vi "reg_check.vi"() -> ()   [LabVIEW 2019]
uses:
  Heating/ctl/ZY_control.ctl
  ctl/Z_State.ctl
  ctl/Y_state.ctl
  Heating/ctl/Z_State.ctl
  Heating/ctl/TMP_val.ctl
  Inputs/Ctl/Parameter State.ctl
  Alarms/Ctl/ALRs_State.ctl
  Alarms/Ctl/ALR_ON_OFF.ctl
  Alarms/Ctl/ALR_Parameters.ctl
  Alarms/Ctl/ALR code.ctl
  Alarms/Ctl/ALR type.ctl
  ctl/ZY_state_short.ctl
  ctl/Z.ctl
  Heating/ctl/Y_source.ctl
  ctl/Y_short.ctl
  ctl/Y_source.ctl
  Inputs/Ctl/Parameter State short.ctl
  Alarms/Ctl/ALR_Status_short.ctl
  ctl/control param.ctl
  projects/Additivs/Regulators/PROG/GM1_201007/HT1/HT1_ALR_on.vi
  Alarms/ALR select.vi
  Alarms/ALR RESETs.vi
  Alarms/ALR ON_OFFs.vi
  bronkhorst_Z.vi
  Heating/Z_switch_heating.vi
  Z_State_reg.vi
  Sequence/State1.vi
  Trigers/RS.vi
  Timer Delay/Timer.vi
  bronkhorst_reg.vi
  Heating/Heating.lvlib
  Alarms/Alarms.lvlib
  Inputs/Inputs.lvlib
  control.lvlib
panel:
  in  "Z_HSw":u32=2
  in  "Y_ASetState":T1=enum."auto"
  out "YB":bool
  out "ALR_L1":bool
  out "Y":dbl format="%.2f"
  out "ZY_State":T2={"Z"={"Z_Source"=enum."initialize", "Z_SetState"=enum."initialization", "Z_State"=enum."initialization", "Z_State_T"=0, "ALR  L1"=FALSE, "ALR  L2"=FALSE, "HH_run"=0}, "Y"={"Y_Source"=enum."initialize", "Y_SetState"=enum."initialize", "SP_Set"=0.0, "SP"=0.0, "PV"=0.0, "PV_State"={"code"=0, "visible"=FALSE, "color"=0}, "Y_preSet"=0.0, "Y_Set"=0.0, "Y"=0.0, "Y_State"={"code"=0, "visible"=FALSE, "color"=0}, "YB"=FALSE}, "ALR_Status"=[], "control param"={"proportional gain (Kc)"=1.0, "integral time (Ti, s)"=10.0, "derivative time (Td, s)"=1.0, "output high"=100.0, "output high start"=40.0, "output high stop"=40.0, "alr value"=0.0, "output low"=0.0, "output rate (EGU/s)"=5.0, "setpoint max"=100.0, "setpoint rate (EGU/min)"=10.0, "stop rate (EGU/min)"=5.0}} {"control param"."setpoint max" format="%.2f"; "control param"."stop rate (EGU/min)" min=0.001 format="%.2f"; "control param"."setpoint rate (EGU/min)" min=0.001 format="%.2f"; "control param"."output high stop" format="%.2f"; "control param"."output high start" format="%.2f"; "control param"."output rate (EGU/s)" min=0.001 format="%.2f"; "control param"."output low" format="%.2f"; "control param"."alr value" format="%.2f"; "control param"."output high" format="%.2f"; "control param"."derivative time (Td, s)" format="%.3f"; "control param"."integral time (Ti, s)" format="%.3f"; "control param"."proportional gain (Kc)" format="%.3f"; "Y"."Y" format="%.2f"; "Y"."Y_preSet" format="%.2f"; "Y"."SP" step=0.01 format="%.2f"; "Y"."Y_Set" format="%.2f"; "Y"."PV" step=0.01 format="%.2f"; "Y"."SP_Set" step=0.01 format="%.2f"}
  in  "TMP_val":T11
  in  "Z_ASetState":T5
  in  "ALR_ON_OFF 2":T18
  in  "ZY_control":T19={"Z_HSw"=2, "Z_HSetState"=enum."initialization", "Y_HSw"=2, "Y_HSetState"=enum."initialize", "SP"=0.0, "Y_H"=0.0, "Reset_ALR"=FALSE} {"Y_H" step=1.0; "SP" step=0.01 format="%.2f"}
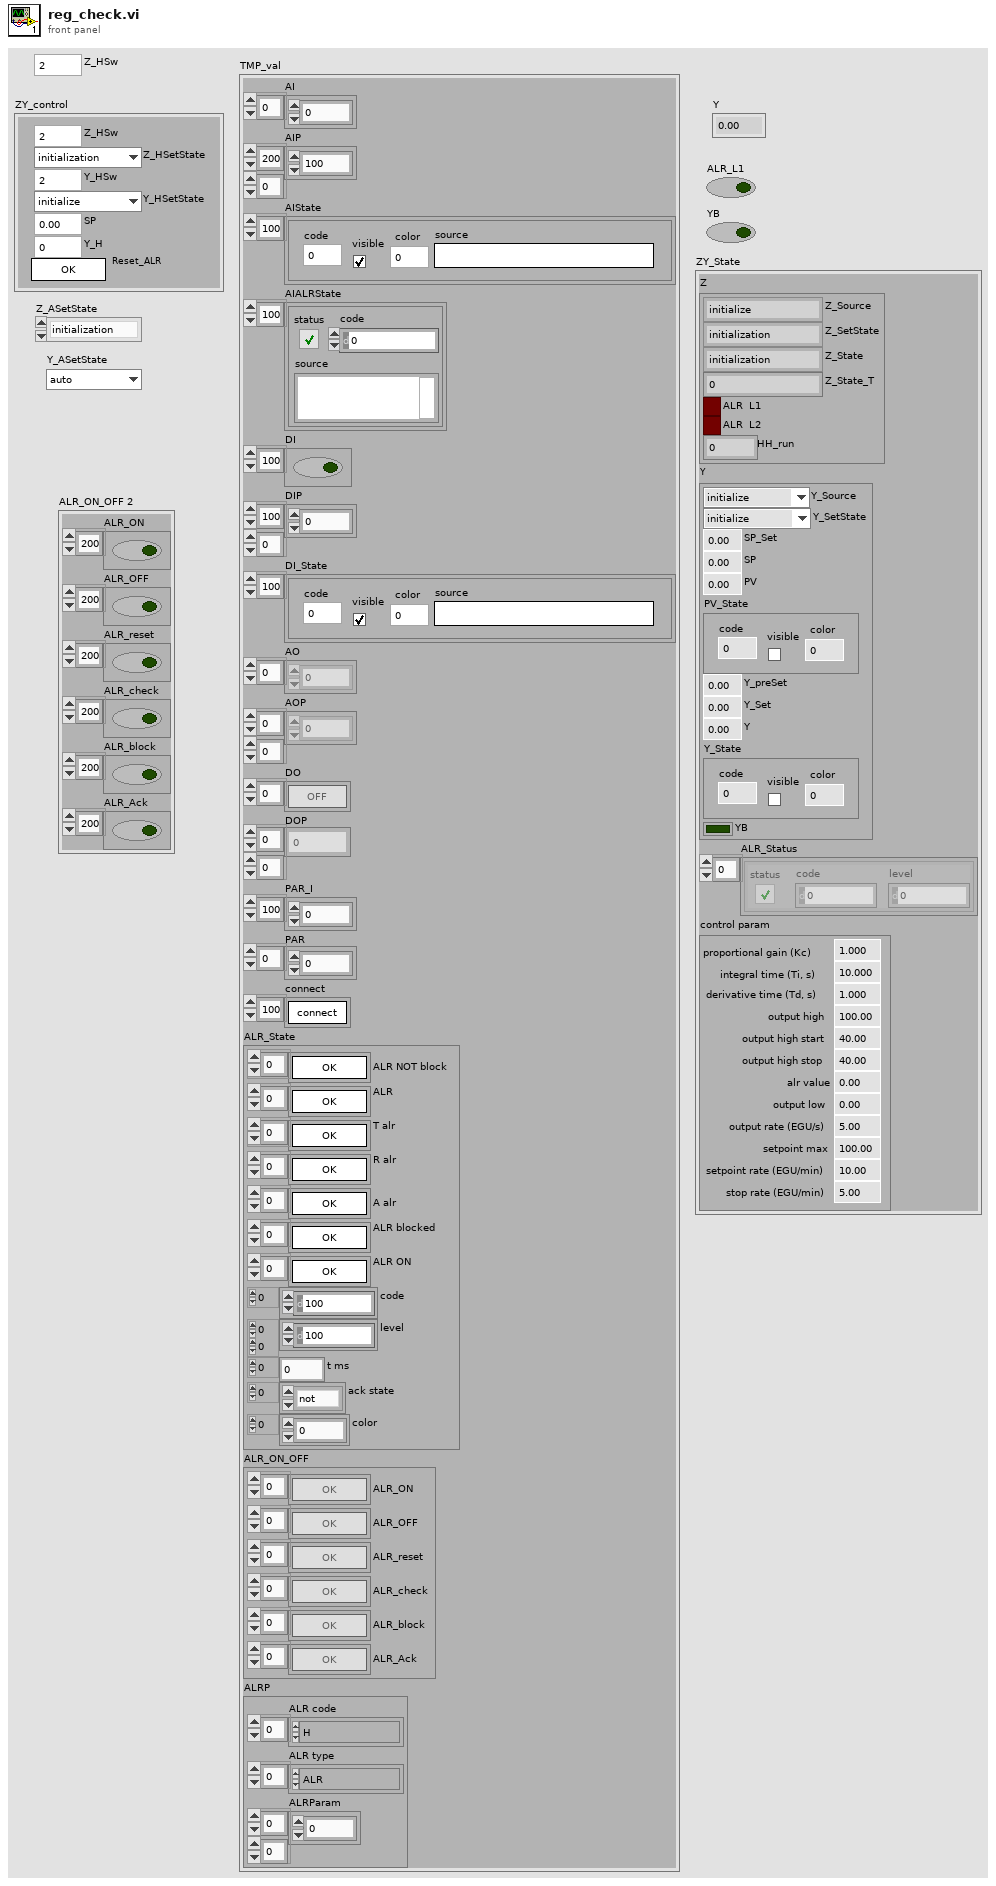
[diagram p1: front panel]
types:
  T1 = typedef "control.lvlib/Y_state.ctl" = enum8{"initialize", "alarm", "min", "stop", "hand", "auto", "max"}
  T2 = typedef "ZY_state_short.ctl" = cluster{"Z":T3, "Y":T6, "ALR_Status":T9[], "control param":T10}
  T3 = typedef "Z.ctl" = cluster{"Z_Source":T4, "Z_SetState":T5, "Z_State":T5, "Z_State_T":u32, "ALR  L1":bool, "ALR  L2":bool, "HH_run":i32}
  T4 = typedef "Heating.lvlib/Y_source.ctl" = enum8{"initialize", "local disabled", "local hand", "hand", "auto", "dist"}
  T5 = typedef "Heating.lvlib/Z_State.ctl" = enum8{"initialization", "alarm", "disabled", "not ready", "stop ready", "reserv", "switched off", "reserv2", "switched on", "check", "on min", "decrease out", "on", "increase out", "on max"}
  T6 = typedef "control.lvlib/Y_short.ctl" = cluster{"Y_Source":T7, "Y_SetState":T1, "SP_Set":dbl, "SP":dbl, "PV":dbl, "PV_State":T8, "Y_preSet":dbl, "Y_Set":dbl, "Y":dbl, "Y_State":T8, "YB":bool}
  T7 = typedef "control.lvlib/Y_source.ctl" = enum8{"initialize", "local disabled", "local hand", "hand", "auto", "dist"}
  T8 = typedef "Inputs.lvlib/Parameter State short.ctl" = cluster{"code":i32, "visible":bool, "color":u32}
  T9 = typedef "Alarms.lvlib/ALR_Status_short.ctl" = cluster{"status":bool, "code":i32, "level":i32}
  T10 = typedef "control param.ctl" = cluster{"proportional gain (Kc)":dbl, "integral time (Ti, s)":dbl, "derivative time (Td, s)":dbl, "output high":dbl, "output high start":dbl, "output high stop":dbl, "alr value":dbl, "output low":dbl, "output rate (EGU/s)":dbl, "setpoint max":dbl, "setpoint rate (EGU/min)":dbl, "stop rate (EGU/min)":dbl}
  T11 = typedef "Heating.lvlib/TMP_val.ctl" = cluster{"AI":dbl[], "AIP":dbl[][], "AIState":T12[], "AIALRState":errorcluster[], "DI":bool[], "DIP":dbl[][], "DI_State":T12[], "AO":dbl[], "AOP":dbl[][], "DO":bool[], "DOP":i32[][], "PAR_I":i32[], "PAR":dbl[], "connect":bool[], "ALR_State":T13, "ALR_ON_OFF":T14, "ALRP":T15}
  T12 = typedef "Inputs.lvlib/Parameter State.ctl" = cluster{"code":i32, "visible":bool, "color":u32, "source":string}
  T13 = typedef "Alarms.lvlib/ALRs_State.ctl" = cluster{"ALR NOT block":bool[], "ALR":bool[], "T alr":bool[], "R alr":bool[], "A alr":bool[], "ALR blocked":bool[], "ALR ON":bool[], "code":i32[], "level":i32[][], "t ms":u32[], "ack state":enum32{"not", "tripped", "reset", "ack"}[], "color":u32[]}
  T14 = typedef "Alarms.lvlib/ALR_ON_OFF.ctl" = cluster{"ALR_ON":bool[], "ALR_OFF":bool[], "ALR_reset":bool[], "ALR_check":bool[], "ALR_block":bool[], "ALR_Ack":bool[]}
  T15 = typedef "Alarms.lvlib/ALR_Parameters.ctl" = cluster{"ALR code":T16[], "ALR type":T17[], "ALRParam":u32[][]}
  T16 = typedef "Alarms.lvlib/ALR code.ctl" = enum16{"CONN", "H", "HH", "L", "LL", "SERR", "ON", "OFF", "XM19", "XM24", "XM47", "XM51", "XM52", "XM53", "XM54", "XM55", "XM56", "XM61", "XM62", "XM63", "XM64", "XM65", "XM66"}
  T17 = typedef "Alarms.lvlib/ALR type.ctl" = enum16{"ACD", "ACDR", "ALRN", "ALR"}
  T18 = cluster{"ALR_ON":bool[], "ALR_OFF":bool[], "ALR_reset":bool[], "ALR_check":bool[], "ALR_block":bool[], "ALR_Ack":bool[]}
  T19 = typedef "Heating.lvlib/ZY_control.ctl" = cluster{"Z_HSw":u32, "Z_HSetState":T20, "Y_HSw":u32, "Y_HSetState":T1, "SP":dbl, "Y_H":dbl, "Reset_ALR":bool}
  T20 = typedef "control.lvlib/Z_State.ctl" = enum8{"initialization", "alarm", "disabled", "not ready", "stop ready", "reserv", "switched off", "reserv2", "switched on", "check", "on min", "decrease out", "on", "increase out", "on max"}
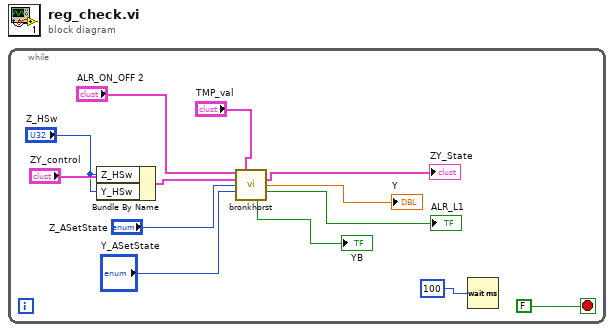
[diagram p0: block diagram]
diagram:
  n1 = while {
    stop <- FALSE stop-if-true
    n2 = Bundle By Name(cluster="ZY_control", "Z_HSw"="Z_HSw", "Y_HSw"="Z_HSw") -> (w2:T19)
    n3 = call "bronkhorst.vi"("ALR_ON_OFF"="ALR_ON_OFF 2", "TMP_val"="TMP_val", "ZY_control"=w2, "Z_ASetState"="Z_ASetState", "Y_ASetState"="Y_ASetState") -> ("ZY_State"=→"ZY_State":T2, "Y"=→"Y":dbl, "ALR_L1"=→"ALR_L1":bool, "YB"=→"YB":bool)  [unwired: 5 in, 2 out]
    n4 = Wait (ms)(milliseconds to wait=u32 100) -> ()  [unwired: 1 out]
  }
